vi "FourierTransform.vi"(1 "Settings":T1={"Name of test"="", "Date"=timestamp(0 s since 1904-01-01), "Location"="", "Template"="", "Soundcard"="", "resolution"=32, "Sampling rate"=48000, "Ch1 Gain "=25.0, "Ch2 Gain"=10.0, "Sample time (s)"=0.3, "Pre-trigger (s)"=0.01, "Hammer Threshold"=10.0, "Positions"=12, "Taps/Position"=5, "Set Names"="", "Freq resolution"=10.0, "Hammer cutoff"=0.0, "Mic cutoff"=0.0, "Double bounce "=0.0, "Hammer Cal"=10.0, "dB Offset"=0.0, "Accel Cal"=10.0, "Vibrometer Cal"=0.0, "Mic Cal"=0.0, "Output"=2, "Voltage Cal"=1.0, "Vibrometer Port"="ASRL27::INSTR", "Range"=4, "High Pass"=2, "Bandwidth"=4, "X Range"=[], "Y Range"=[], "dB Spread"=0.0, "Trigger"=0, "Ch_1"=25, "Ch_2"=25, "flip?"=FALSE, "60Hz"=FALSE, "Time offset"=0.0, "Piezo Cal"=1.0, "Default Notes"=""} {"Ch_2" min=1 step=1; "Ch_1" min=1 max=100 step=1; "Trigger" items=["Hammer (force)", "Self-tap", "Spacebar"]; "Bandwidth" items=["1 kHz"=1, "5 kHz"=5, "10 kHz"=10, "25 kHz"=25, "50 kHz"=50, "100 kHz"=100]; "High Pass" items=["Off", "13 Hz", "104 Hz"]; "Range" items=["10 mm/s"=1, "20 mm/s"=2, "50 mm/s"=5, "100 mm/s"=10, "200 mm/s"=20, "500 mm/s"=50, "1 m/s"=100, "2 m/s"=200]; "Output" items=["Accelerometer", "Speed (from acceleration)", "Microphone", "Vibrometer", "Piezo"]; "Voltage Cal" format="%#_13g"; "Ch2 Gain" format="%#_13g"; "Ch1 Gain" format="%#_13g"; "Double bounce" min=0.0; "Mic cutoff" min=0.0 format="%#_4g"; "Hammer cutoff" min=0.0 format="%#_4g"; "Freq resolution" min=0.0; "Pre-trigger (s)" format="%#_13g"; "Date" format="%<%H:%M\n%d/%m/%y>T"; "resolution" items=["16 bit"=16, "24 bit"=24, "32 bit"=32]; "Sampling rate" items=["22050 samp/s"=22050, "44100 samp/s"=44100, "48000 samp/s"=48000]}, 3 "Data":waveform(dbl)(graph)) -> (2 "Magnitude of Spectrum":cluster{"x0":dbl, "df":dbl, dbl[]}(graph), 5 "FFT":cluster{dbl, "df":dbl, "FFT {X}":cdb[]})   [LabVIEW 2022 SP3]
uses:
  PreferencesControl.ctl
  <vilib>/Analysis/2dsp.llb/Real FFT.vi
  <vilib>/Analysis/NI_AALPro.lvlib
panel:
  # "Hz"
  # "dB"
  # "dB"
  # "sec"
  # "sec"
  # "mV/Pa"
  # "mV/m/s2"
  # "mV/mm/s"
  # "V/N"
  # "sec"
  # "sec"
  # "mV/N"
  # "a.u."
  # "a.u."
  # "sec"
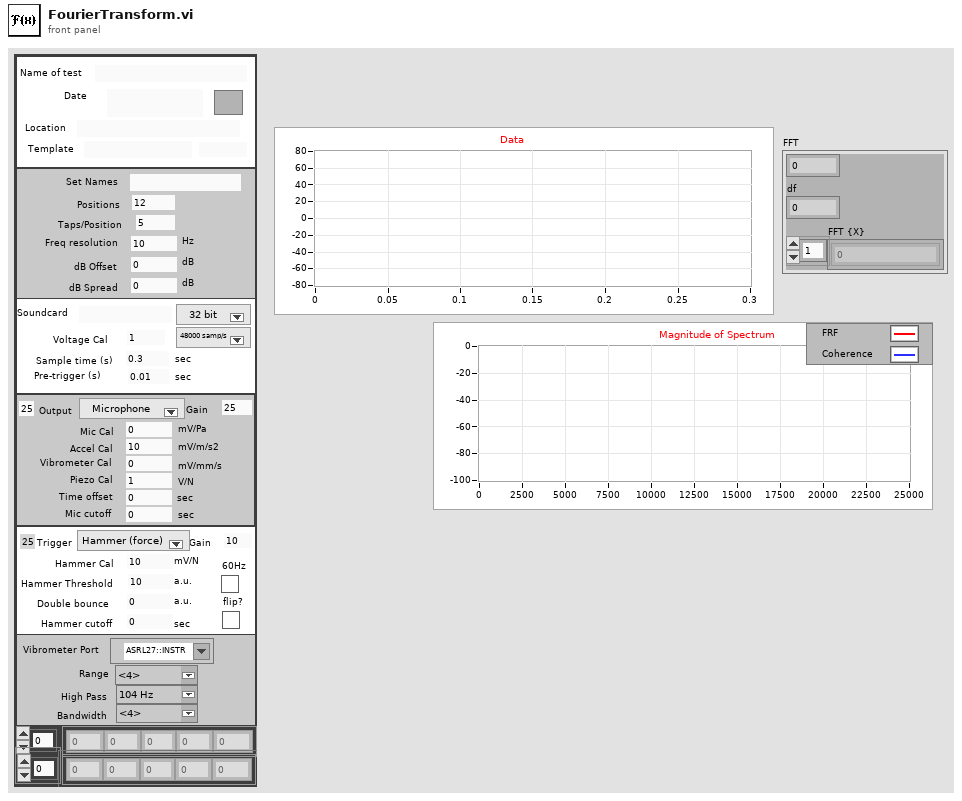
[diagram p1: front panel]
types:
  T1 = typedef "PreferencesControl.ctl" = cluster{"Name of test":string, "Date":timestamp, "Location":string, "Template":string, "Soundcard":string, "resolution":u16, "Sampling rate":u16, "Ch1 Gain ":dbl, "Ch2 Gain":dbl, "Sample time (s)":dbl, "Pre-trigger (s)":dbl, "Hammer Threshold":dbl, "Positions":i16, "Taps/Position":i16, "Set Names":string, "Freq resolution":dbl, "Hammer cutoff":dbl, "Mic cutoff":dbl, "Double bounce ":dbl, "Hammer Cal":dbl, "dB Offset":dbl, "Accel Cal":dbl, "Vibrometer Cal":dbl, "Mic Cal":dbl, "Output":u16, "Voltage Cal":dbl, "Vibrometer Port":refnum<visa-resource-name>, "Range":u16, "High Pass":u16, "Bandwidth":u16, "X Range":cluster{"Minimum":dbl, "Maximum":dbl, "Increment":dbl, "Minor Increment":dbl, "Start":dbl}[], "Y Range":cluster{"Minimum":dbl, "Maximum":dbl, "Increment":dbl, "Minor Increment":dbl, "Start":dbl}[], "dB Spread":dbl, "Trigger":u16, "Ch_1":u8, "Ch_2":u8, "flip?":bool, "60Hz":bool, "Time offset":dbl, "Piezo Cal":dbl, "Default Notes":string}
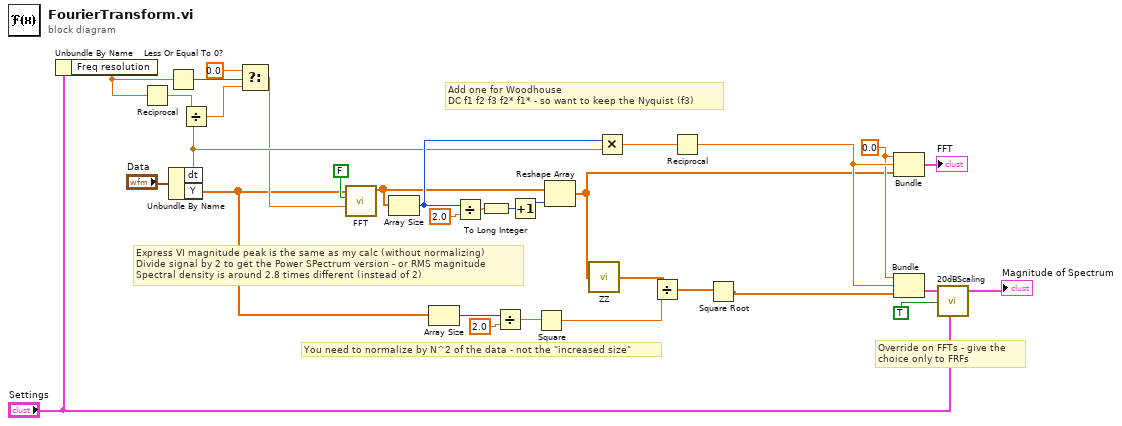
[diagram p0: block diagram]
diagram:
  w11 = 0.0 ("t")
  # "Add one for Woodhouse\nDC f1 f2 f3 f2* f1* - so want to keep the Nyquist (f3)"
  # "You need to normalize by N^2 of the data - not the \"increased size\""
  # "Override on FFTs - give the \nchoice only to FRFs"
  # "Express VI magnitude peak is the same as my calc (without normalizing)\nDivide signal by 2 to get the Power SPectrum version - or RMS magnitude\nSpectral density is around 2.8 times different (instead of 2)"
  n1 = Unbundle By Name("Settings") -> ("Freq resolution"=w12:dbl)
  n2 = Reciprocal(x=w12) -> (1/x=w23:dbl)
  n3 = Less Or Equal To 0?(x=w12) -> (x <= 0?=w16:bool)
  n4 = Unbundle By Name("Data") -> ("dt"=w22:dbl, "Y"=w3:dbl[])
  n5 = Divide(x=w23, y=w22) -> (x/y=w19:dbl)
  n6 = Select(t=0.0, s=w16, f=w19) -> (s? t:f=w17:dbl)
  n7 = call-poly <vilib>:"FFT.vi"("FFT size"=w17, "shift?"=FALSE, "X"=w3) -> ("FFT {X}"=w25:cdb[])  [unwired: 7 in, 1 out]
  n8 = Array Size(array=w25) -> (size(s)=w26:i32)
  n9 = Array Size(array=w3) -> (size(s)=w5:i32)
  n10 = Divide(x=w26, y=2.0) -> (x/y=w29:dbl)
  n11 = To Long Integer(number=w29) -> (32bit integer=w30:i32)
  n12 = Divide(x=w5, y=2.0) -> (x/y=w2:dbl)
  n13 = Increment(x=w30) -> (x+1=w1:i32)
  n14 = Square(x=w2) -> (x^2=w9:dbl)
  n15 = Reshape Array(w25, w1) -> (w7:cdb[])
  n16 = call "ZZ.vi"("P"=w7) -> ("PP*"=w10:dbl[])
  n17 = Multiply(x=w26, y=w22) -> (x*y=w27:dbl)
  n18 = Divide(x=w10, y=w9) -> (x/y=w8:dbl[])
  n19 = Reciprocal(x=w27) -> (1/x=w14:dbl)
  n20 = Square Root(x=w8) -> (sqrt(x)=w6:dbl[])
  n21 = Bundle("t"=w11, w14, "FFT {X}"=w7) -> (→"FFT":cluster{"t":dbl, dbl, "FFT {X}":cdb[]})  [unwired: 1 in]
  n22 = Bundle("t"=w11, w14, w6) -> (w21:cluster{"t":dbl, dbl, dbl[]})  [unwired: 1 in]
  n23 = call "20dBScaling.vi"("Average FRF in"=w21, "dB?"=TRUE, "Settings"="Settings") -> ("Average FRF out"=→"Magnitude of Spectrum":cluster{"x0":dbl, "df":dbl, dbl[]})  [unwired: 3 in, 1 out]
